vi "logging.vi"(1 "data":string, 2 "Boolean":bool) -> ()   [LabVIEW 2011]
uses:
  <vilib>/Utility/file.llb/Write To Spreadsheet File (string).vi
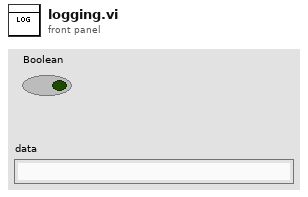
[diagram p1: front panel]
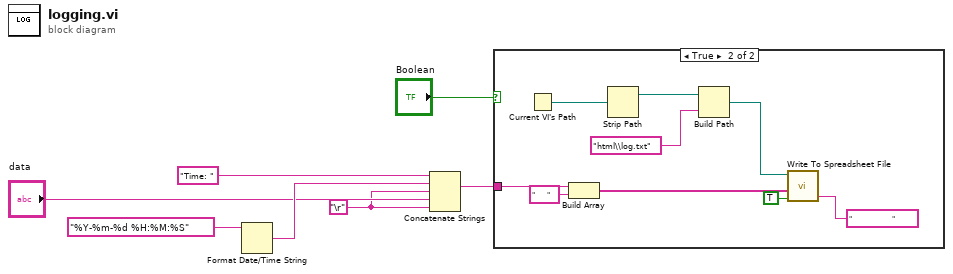
[diagram p0: block diagram]
diagram:
  w1 = "\r"
  n1 = Format Date/Time String(time format string (%c)="%Y-%m-%d %H:%M:%S") -> (date/time string=w4:string)  [unwired: 2 in]
  n2 = Concatenate Strings("Time: ", w4, w1, "data", w1) -> (w2:string)
  n3 = case shown="True" "Boolean" {
    tunnel: w2 -> [_ w9]
    frame False {
    }
    frame True {
      n4 = Current VI's Path() -> (path=w14:path)
      n5 = Build Array(w9, "      " ("element")) -> (w10:string[])
      n6 = Strip Path(path=w14) -> (stripped path=w13:path)  [unwired: 1 out]
      n7 = Build Path(base path=w13, name or relative path="html\\log.txt") -> (appended path=w15:path)
      n8 = call-poly <vilib>:"Write To Spreadsheet File.vi"("delimiter (\\t)"="                    ", "append to file? (new file:F)"=TRUE, "1D data"=w10, "file path (dialog if empty)"=w15) -> ()  [unwired: 4 in, 1 out]
    }
  }
